vi "MQTT Subscriber.vi"() -> ()   [LabVIEW 2021]
uses:
  <vilib>/LabVIEW Open Source Project/MQTT Control Packets/Control Packets/CONNECT/ConnectFlags -- cluster.ctl
  <vilib>/LabVIEW Open Source Project/MQTT Client/Client class/Client.lvclass/Client.ctl
  <vilib>/LabVIEW Open Source Project/MQTT Client/Client class/Client.lvclass
  C:/Program Files (x86)/National Instruments/LabVIEW 2021/vi.lib/LabVIEW Open Source Project/MQTT Connection/MQTT_Base/Base Class/MQTT_Base.lvclass
  <vilib>/LabVIEW Open Source Project/Connection/Connection.TCP/Connection.TCP.lvclass
  C:/Program Files (x86)/National Instruments/LabVIEW 2021/vi.lib/LabVIEW Open Source Project/Connection/Connection/Connection.lvclass
  <vilib>/LabVIEW Open Source Project/MQTT Control Packets/Control Packets/PUBLISH/PUBLISH.lvclass
  <vilib>/LabVIEW Open Source Project/MQTT Connection/MQTT_Base/Base Class/MQTT_Base.lvclass
  <vilib>/LabVIEW Open Source Project/MQTT Control Packets/Control Packets/CONNECT/CONNECT.lvclass
panel:
  out "Connected?":bool
  out "Data Chart":dbl(graph)
  out "Data":dbl format="%#_4g"
  in  "Topic":string
  in  "remote port (1883)":u16=1883
  in  "address (localhost)":string="localhost"
  in  "STOP":bool
  # "MQTT Subscriber"
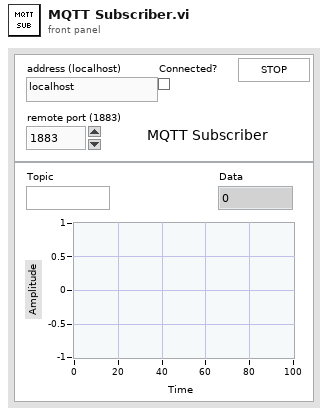
[diagram p1: front panel]
types:
  T1 = enum32{"Invalid", "Standard", "Closed", "Hidden", "Minimized", "Maximized"}
  T2 = enum32{"invalid app kind", "Development System", "Run Time System", "Student Edition", "Embedded LabVIEW", "Evaluation", "Custom"}
  T3 = cluster{"Will Topic":string, "Will Message":string, "Username":string, "Password":string}
  T4 = typedef "MQTT_Control_Packets.lvlib/CONNECT.lvclass/ConnectFlags -- cluster.ctl" = cluster{"Reserved":bool, "Clean Session":bool, "Will Flag":bool, "Will QoS 1":bool, "Will QoS 2":bool, "Will Retain":bool, "Password Flag":bool, "User Name Flag":bool}
  T5 = cluster{"Core":cluster{"Current VI Reference":refnum<vi>, "Close Panel on Exit?":bool}, "Connected?":bool}
  T6 = cluster{"Current VI Reference":refnum<vi>, "Close Panel on Exit?":bool}
  T7 = typedef "MQTT Client.lvlib/Client.lvclass/Public Events -- cluster.ctl" = cluster{"Connection Status":refnum<user-event>, "Connected":refnum<user-event>, "Application Message":refnum<user-event>}
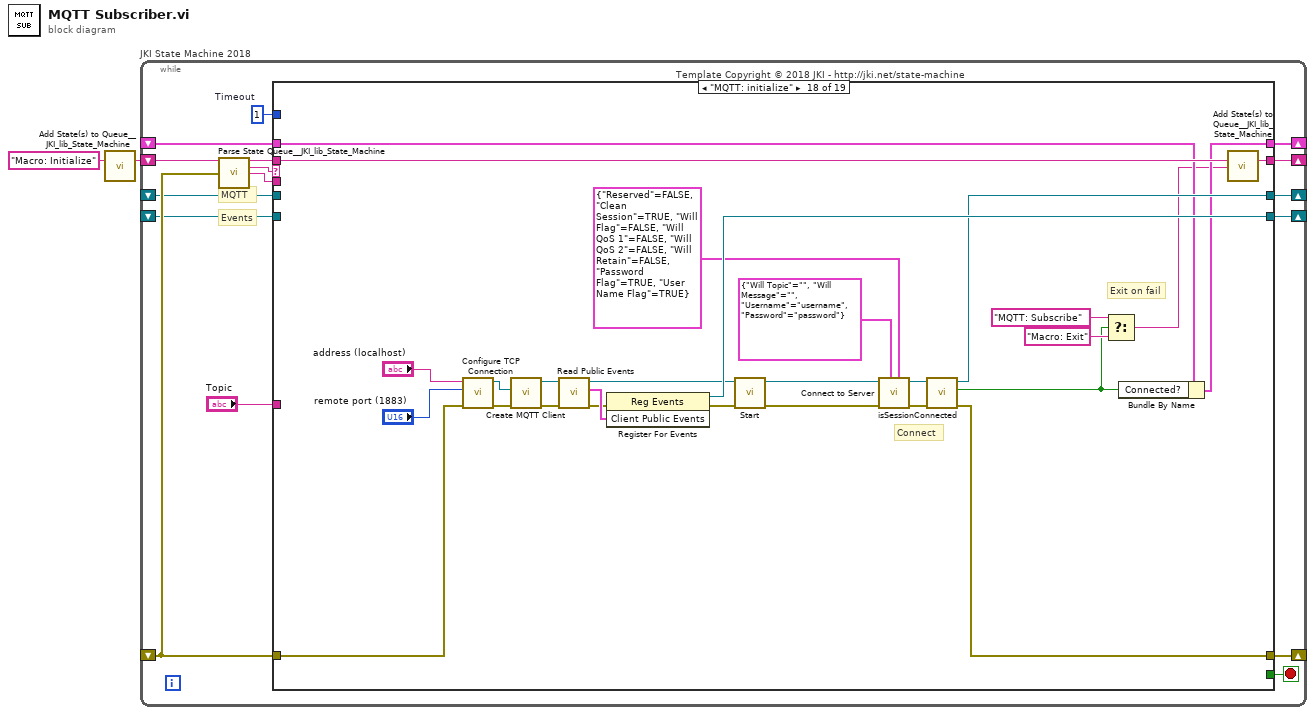
[diagram p0: block diagram]
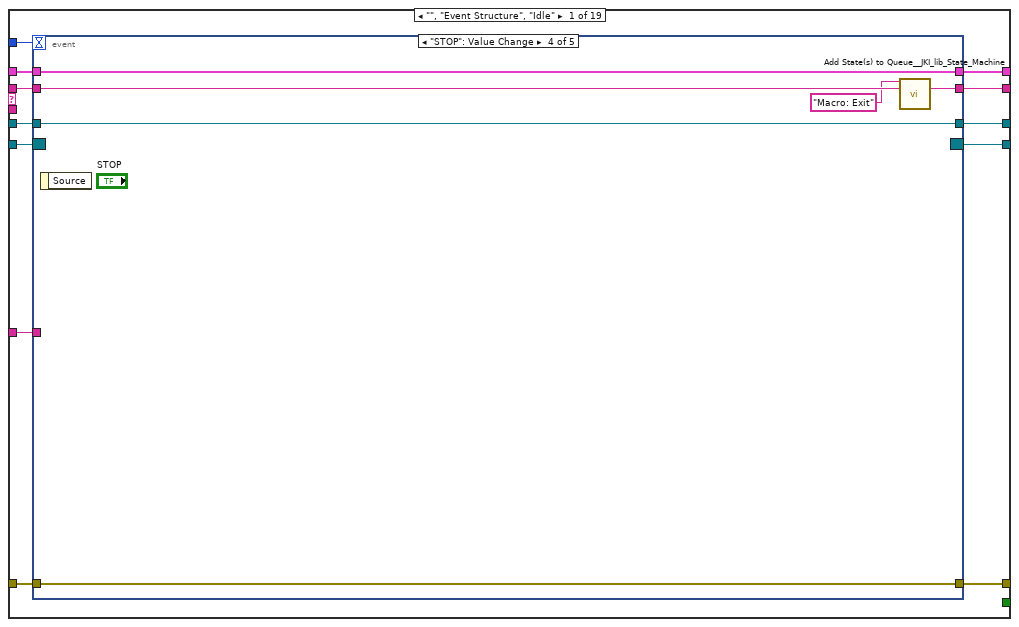
[diagram p2: hidden frame]
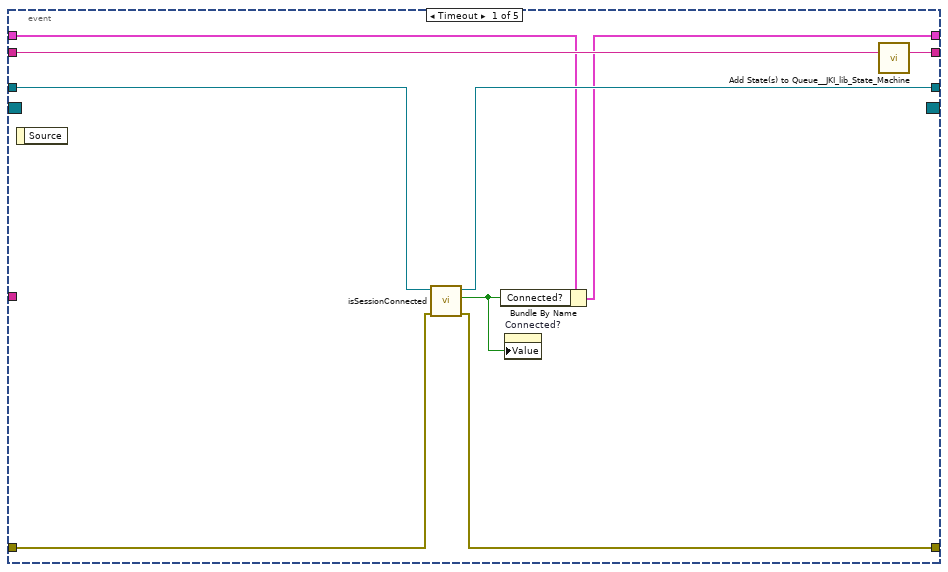
[diagram p3: hidden frame]
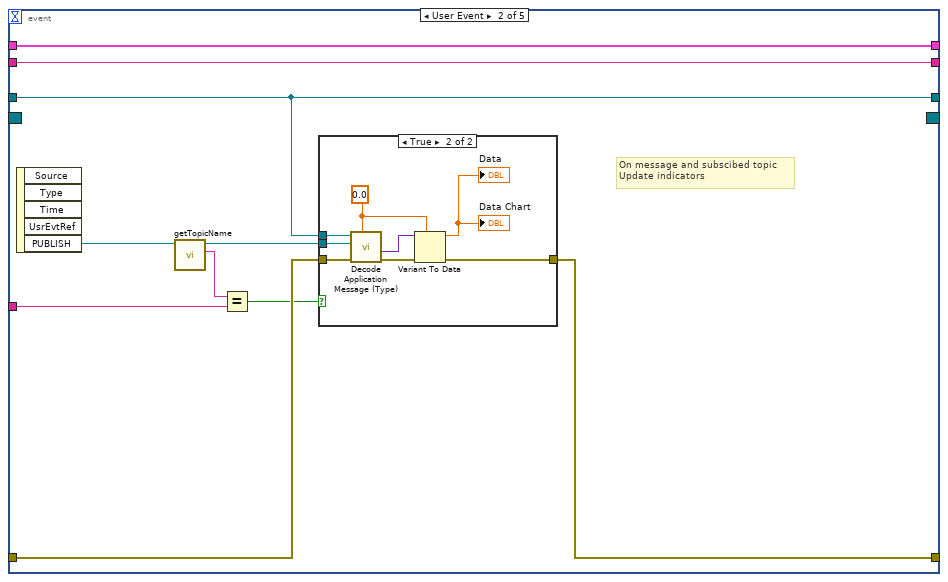
[diagram p4: hidden frame]
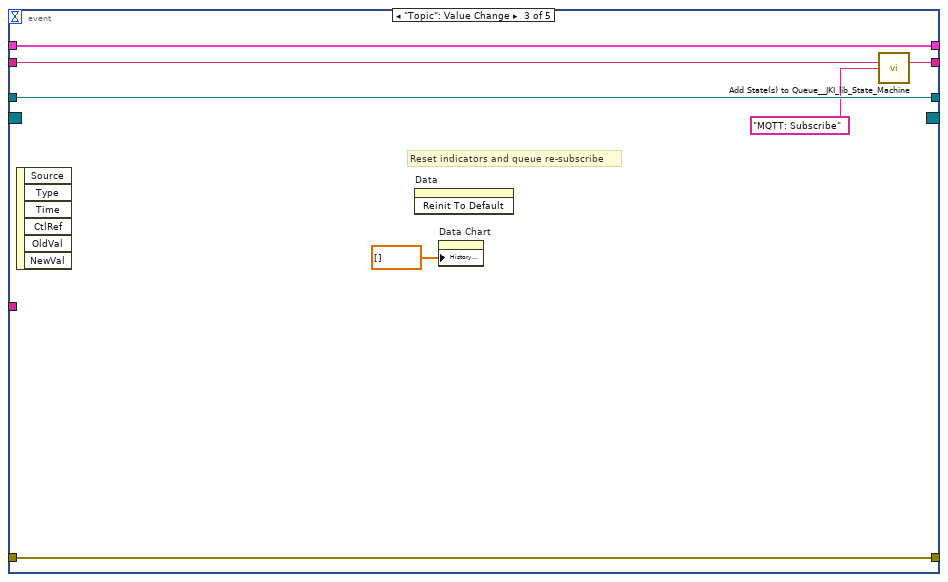
[diagram p6: hidden frame]
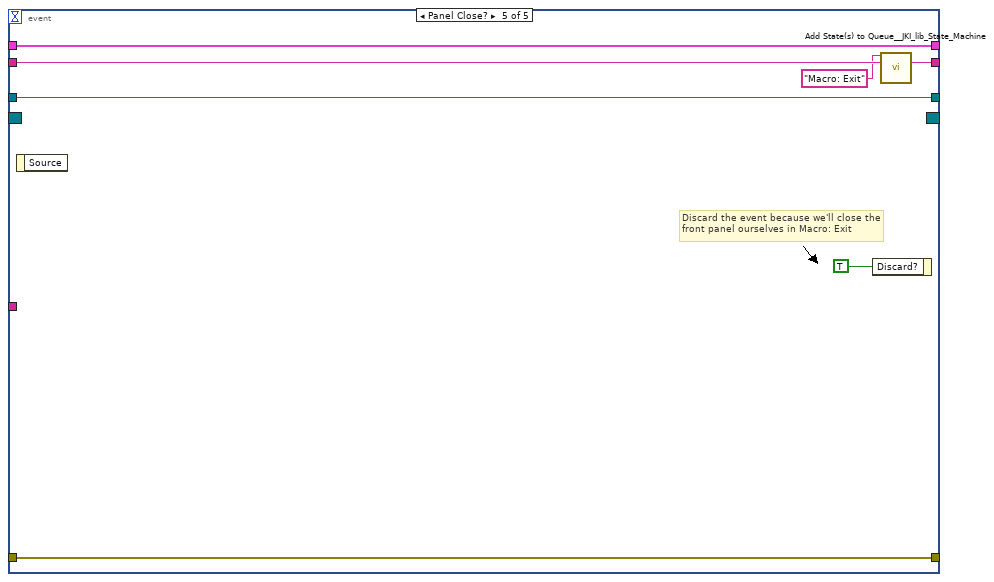
[diagram p7: hidden frame]
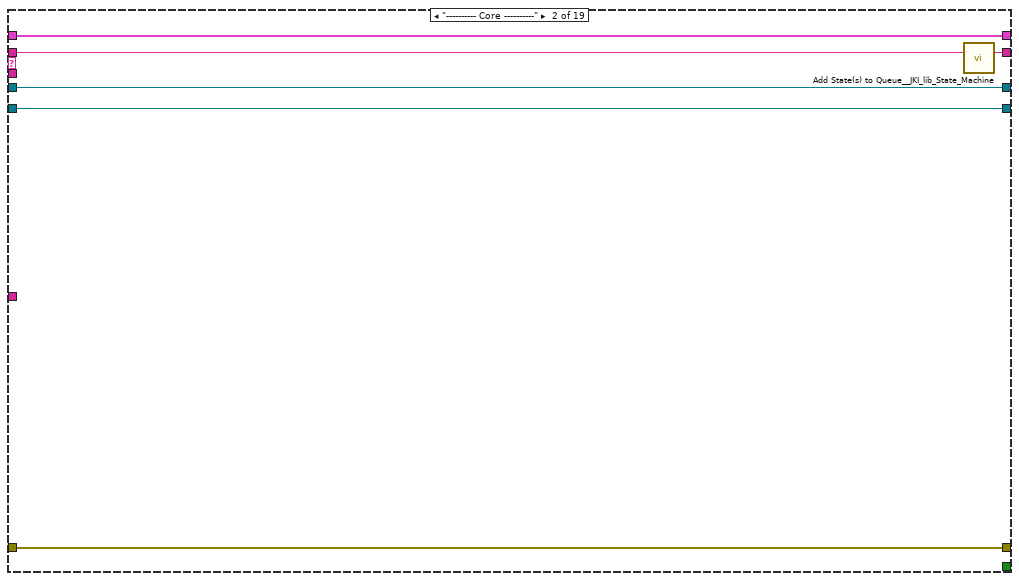
[diagram p8: hidden frame]
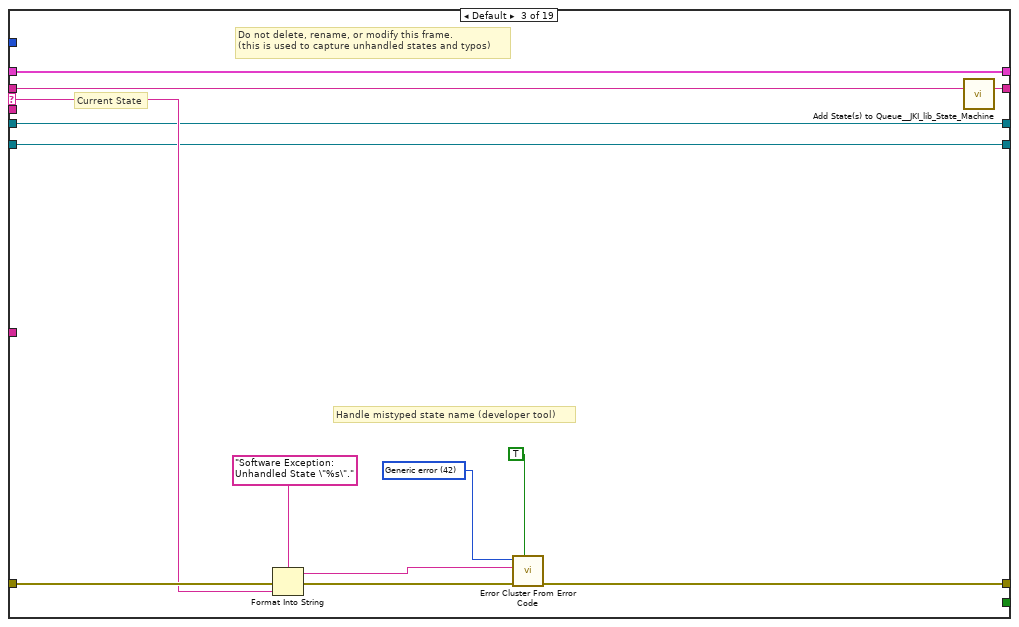
[diagram p9: hidden frame]
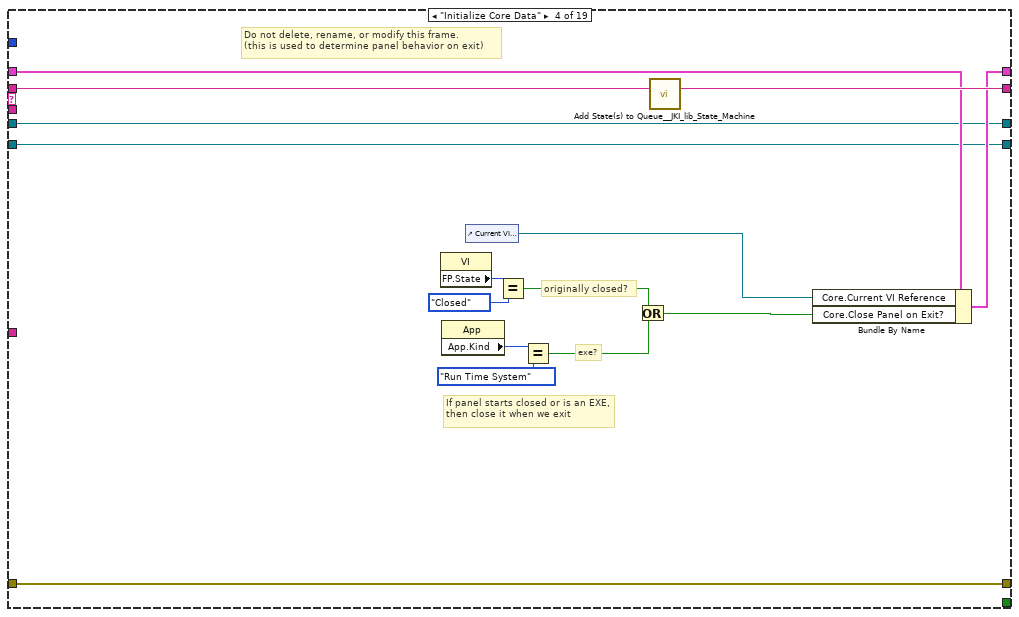
[diagram p10: hidden frame]
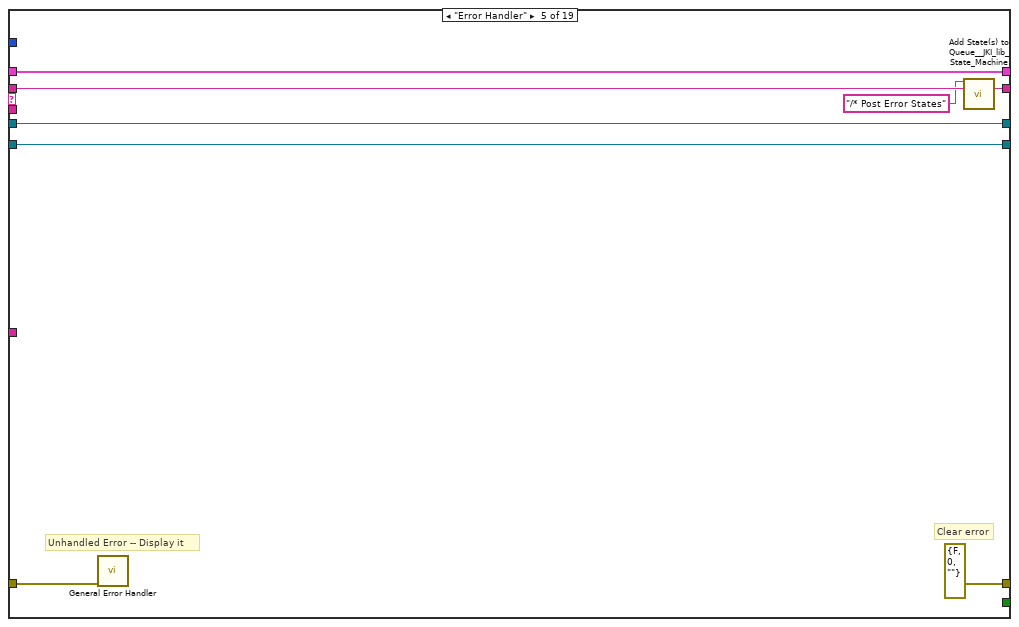
[diagram p11: hidden frame]
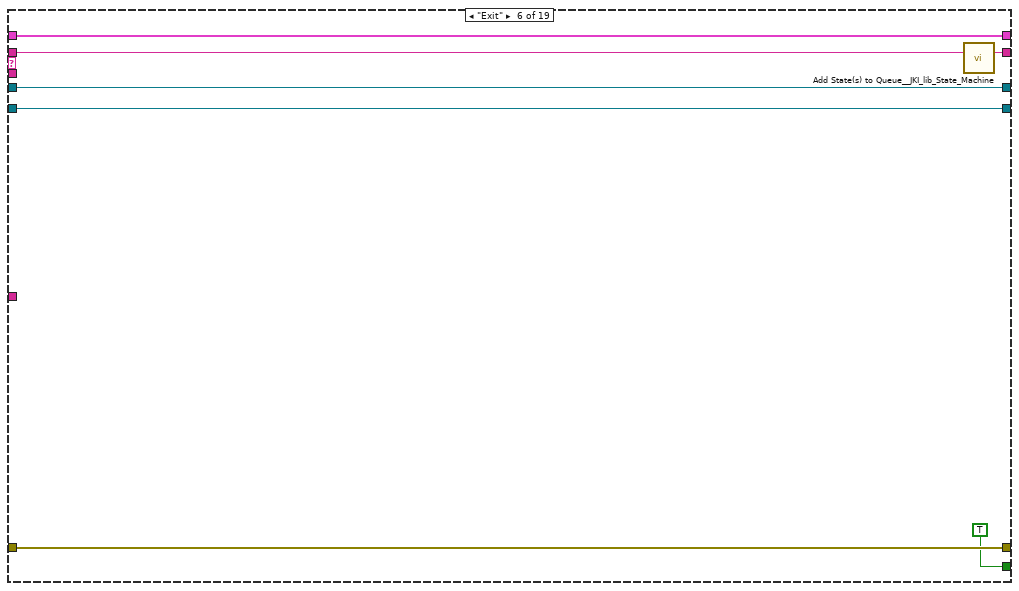
[diagram p12: hidden frame]
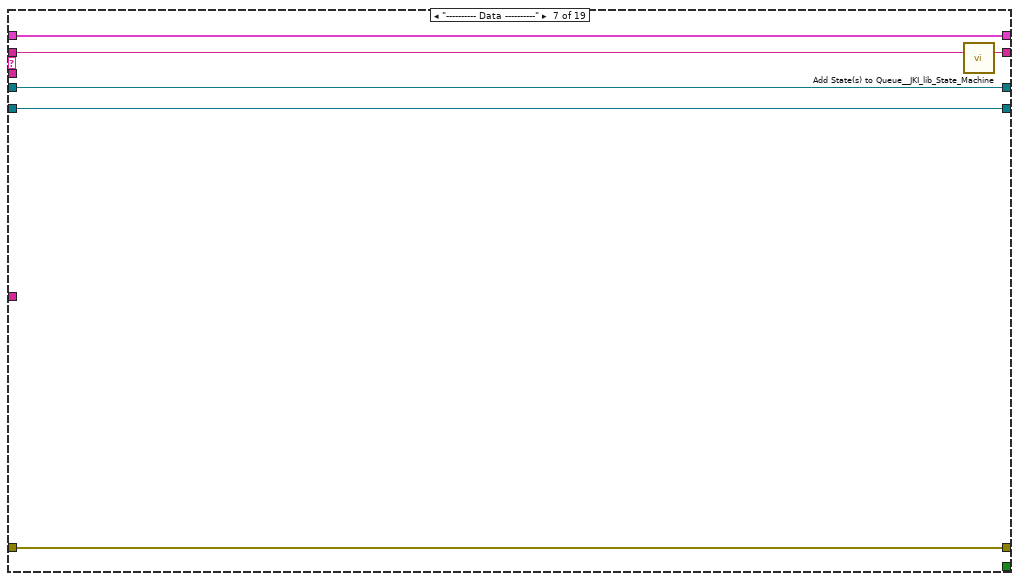
[diagram p13: hidden frame]
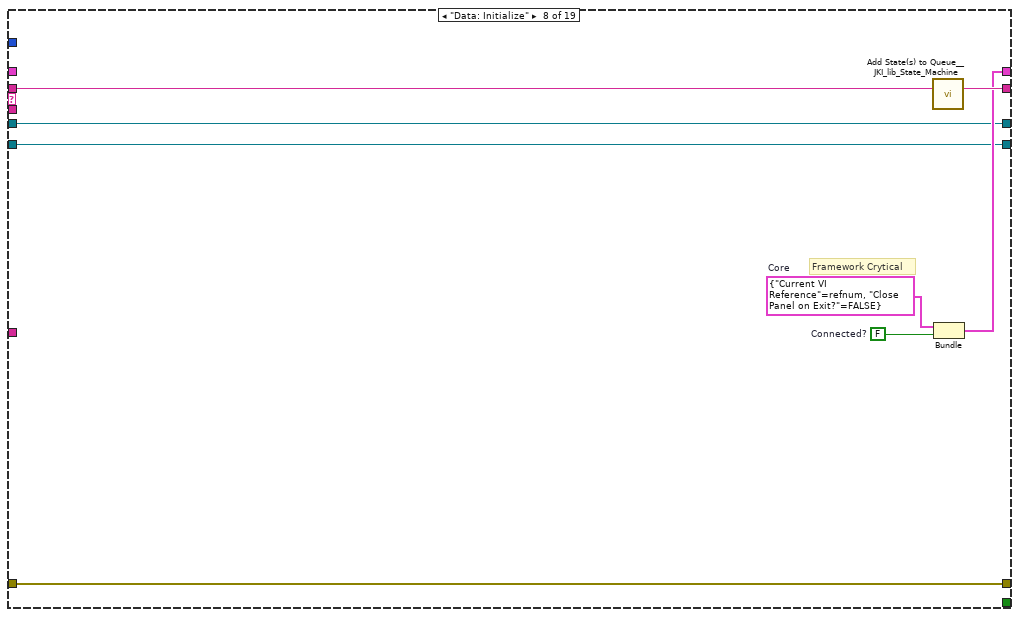
[diagram p14: hidden frame]
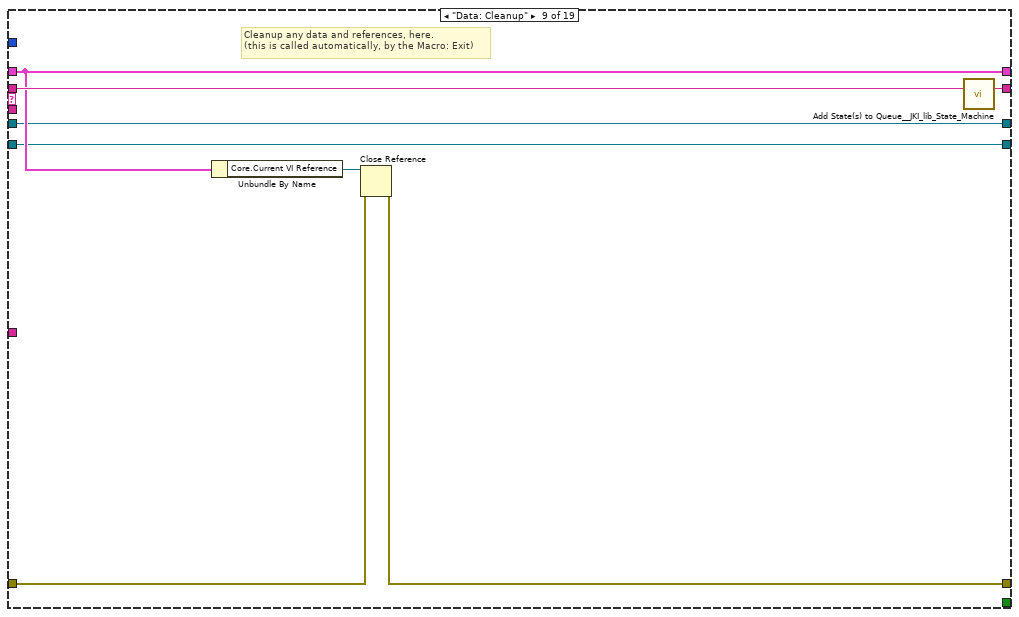
[diagram p15: hidden frame]
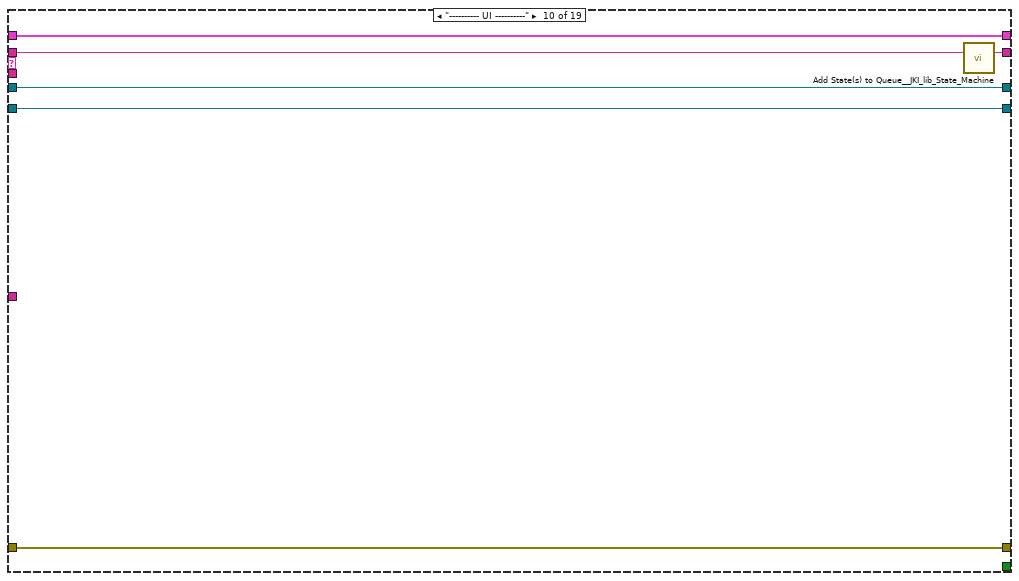
[diagram p16: hidden frame]
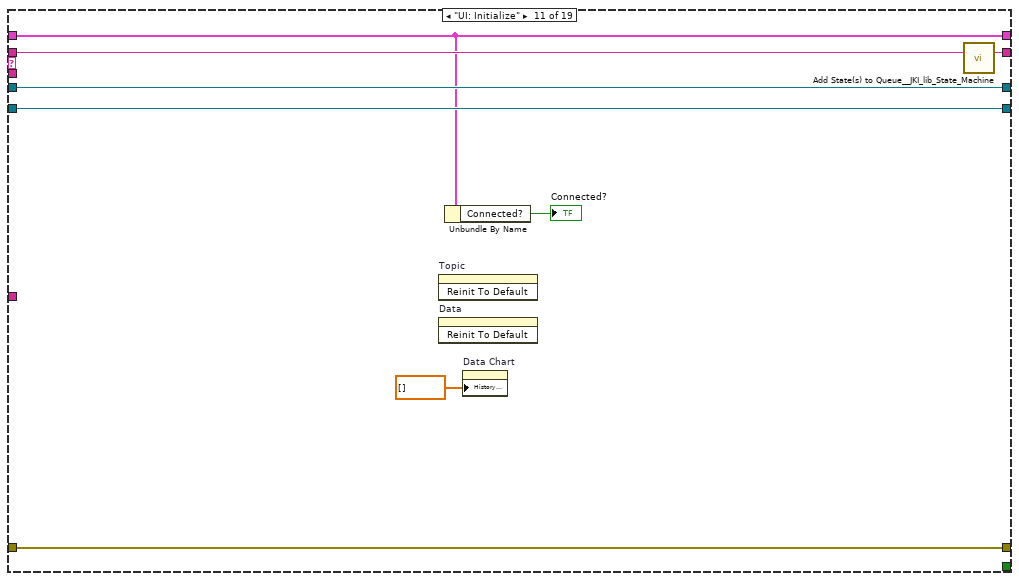
[diagram p17: hidden frame]
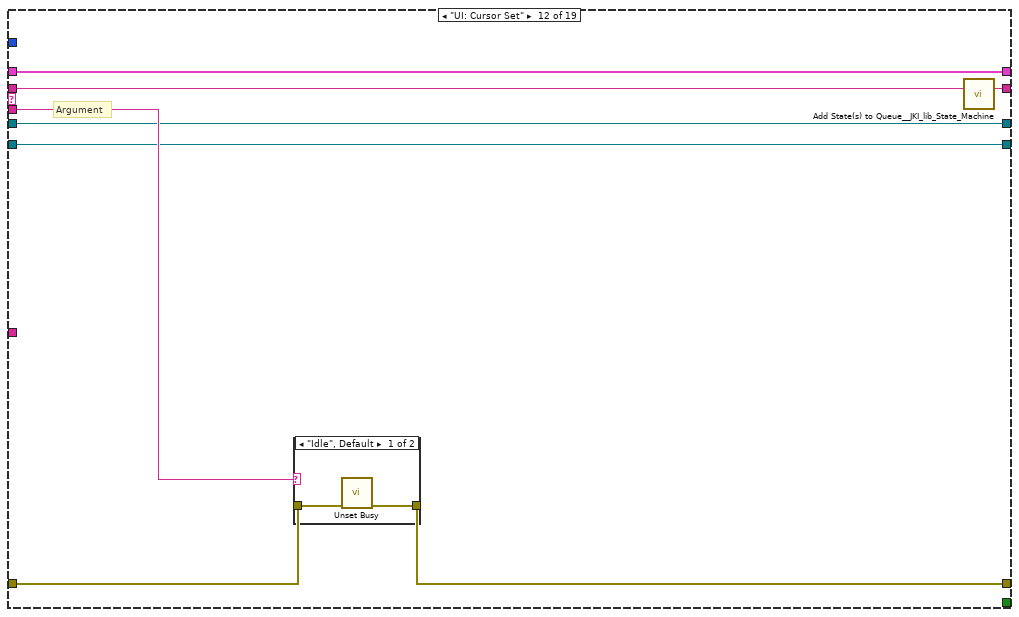
[diagram p18: hidden frame]
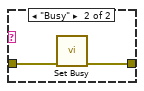
[diagram p19: hidden frame]
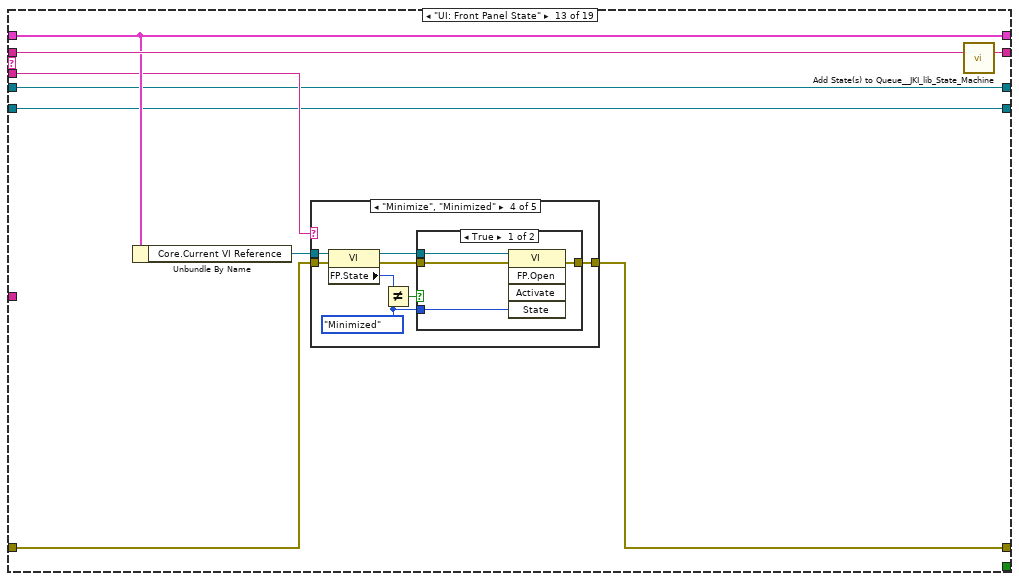
[diagram p20: hidden frame]
diagram:
  n1 = call <vilib>:"Add State(s) to Queue__JKI_lib_State_Machine.vi"("State(s) in (\"\")"="Macro: Initialize") -> ("States Out"=w2:string)  [unwired: 14 in]
  n2 = while "JKI State Machine 2018" {
    shift-right: [w11] -> _
    shift-left: _ -> [w10]
    shift-right: [w14] -> _
    shift-left: _ -> [w8]
    shift-right: [w13] -> _
    shift-left: w2 -> [w15]
    shift-right: [w7] -> _
    shift-left: _ -> [w6]
    shift-right: [w5] -> _
    shift-left: _ -> [w4]
    stop <- w12 stop-if-true
    w9 = 1  # Timeout
    # "Events"
    # "MQTT"
    # "Template Copyright © 2018 JKI - http://jki.net/state-machine"
    n3 = call <vilib>:"Parse State Queue__JKI_lib_State_Machine.vi"("State Queue"=w15, "Error In (no error)"=w8) -> ("Remaining States"=w17:string, "Current State"=w18:string, "Arguments"=w16:string)  [unwired: 11 in]
    n4 = case shown="\"MQTT: initialize\"" w18 {
      selector: w18 -> [_ _ w87 _ _ _ _ _ _ _ _ _ _ _ _ _ _ _ _]
      tunnel: w17 -> [w30 w84 w91 w112 w120 w127 w133 w141 w149 w155 w163 w171 w184 w255 w262 w274 w280 w308 w310]
      tunnel: w16 -> [_ _ _ _ _ _ _ _ _ _ _ w166 w178 _ _ _ _ _ _]
      tunnel: w10 -> [w28 w81 w89 w105 w117 w125 w130 _ w144 w152 w158 w169 w180 w252 w259 w271 w277 w288 w309]
      tunnel: [w27 w82 w93 w109 errorcluster {"status"=FALSE, "code"=0, "source"=""} ("error out") w124 w131 w138 w145 w153 w161 w167 w181 w253 w260 w272 w278 w290 w311] -> w14
      tunnel: w8 -> [w26 w82 w92 w109 w116 w124 w131 w138 w146 w153 w161 w168 w182 w253 w260 w272 w278 w306 w312]
      tunnel: [w29 w83 w90 w111 w119 w126 w132 w140 w148 w154 w162 w170 w183 w254 w261 w273 w279 w307 w310] -> w13
      tunnel: [_ _ _ _ _ TRUE _ _ _ _ _ _ _ _ _ _ _ _ _] -> w12
      tunnel: [w25 w81 w89 w110 w117 w125 w130 w139 w144 w152 w158 w169 w180 w252 w259 w271 w277 w287 w309] -> w11
      tunnel: w9 -> [w24 _ _ _ _ _ _ _ _ _ _ _ _ _ _ _ _ _ _]
      tunnel: [w20 w79 w85 w98 w113 w121 w128 w134 w142 w150 w159 w164 w176 w250 w256 w263 w275 w305 w319] -> w7
      tunnel: w6 -> [w21 w79 w85 w98 w113 w121 w128 w134 w142 w150 w159 w164 w176 w250 w256 w263 w275 _ w319]
      tunnel: [w22 w80 w86 w99 w114 w122 w129 w135 w143 w151 w160 w165 w177 w251 w257 w264 w276 w289 w313] -> w5
      tunnel: w4 -> [w23 w80 w86 w99 w114 w122 w129 w135 w143 w151 w160 w165 w177 w251 w257 w264 w276 _ w314]
      tunnel: "Topic" -> [w19 _ _ _ _ _ _ _ _ _ _ _ _ _ _ _ _ _ w315]
      frame "", "Event Structure", "Idle" {
        n5 = event shown="[3] \"STOP\": Value Change" {
          selector: w21 -> [_ _ _ _ _]
          dyn-events: [_ _ _ _ _] -> w20
          timeout: w24 -> [_ _ _ _ _]
          tunnel: w30 -> [w39 w49 w64 w71 w78]
          tunnel: [w38 w49 w63 w70 w77] -> w29
          tunnel: w28 -> [w33 w48 w65 w68 w75]
          tunnel: [w34 w42 w62 w69 w76] -> w27
          tunnel: w26 -> [w35 w43 w62 w69 w76]
          tunnel: [w32 w48 w65 w68 w75] -> w25
          tunnel: w23 -> [w37 w44 w61 w66 w72]
          tunnel: [w36 w44 w61 w66 w72] -> w22
          tunnel: w19 -> [_ w45 _ _ _]
          event Timeout {
            n6 = event-data() -> ()  [unwired: 1 in, 1 out]
            n7 = call <vilib>:"isSessionConnected.vi"("error in (no error)"=w35, "MQTT_Base in"=w37) -> ("error out"=w34:errorcluster, "Connected?"=w31:bool, "MQTT_Base out"=w36:refnum<class "Client.lvclass">)  [unwired: 7 in]
            n8 = Bundle By Name(cluster=w33, "Connected?"=w31) -> (w32:T5)
            n9 = property on="Connected?" class="Bool (strict)"("Value"=w31) -> ()  [unwired: 2 in, 2 out]
            n10 = call <vilib>:"Add State(s) to Queue__JKI_lib_State_Machine.vi"("State(s) in (\"\")"=w39) -> ("States Out"=w38:string)  [unwired: 14 in]
          }
          event User Event {
            # "On message and subscibed topic\nUpdate indicators"
            n11 = event-data() -> ("PUBLISH"=w47:refnum<class "PUBLISH.lvclass">)  [unwired: 1 in, 4 out]
            n12 = call <vilib>:"getTopicName.vi"("PUBLISH in"=w47) -> ("Topic"=w46:string, "PUBLISH out"=w40:refnum<class "PUBLISH.lvclass">)  [unwired: 8 in, 1 out]
            n13 = Equal?(x=w46, y=w45) -> (x = y?=w41:bool)
            n14 = case shown="True" w41 {
              tunnel: w44 -> [_ w58]
              tunnel: w43 -> [w50 w57]
              tunnel: [w50 w52] -> w42
              tunnel: w40 -> [_ w51]
              frame False {
              }
              frame True {
                w54 = 0.0
                n15 = call <vilib>:"Decode Application Message (Type).vi"("Type"=w54, "error in (no error)"=w57, "PUBLISH"=w51, "Client in"=w58) -> ("error out"=w55:errorcluster, "Payload"=w56:variant)  [unwired: 4 in, 2 out]
                n16 = Variant To Data(error in=w55, type=w54, Variant=w56) -> (data=→"Data" →"Data Chart":dbl, error out=w52:errorcluster)
              }
            }
          }
          event "Topic": Value Change {
            # "Reset indicators and queue re-subscribe"
            n17 = event-data() -> ()  [unwired: 1 in, 6 out]
            n18 = invoke on="Data" class="DigNum (strict)" method="Reinit To Default"() -> ()  [unwired: 3 in, 3 out]
            n19 = property on="Data Chart" class="WFChart (strict)"("History Data"=dbl[] []) -> ()  [unwired: 2 in, 2 out]
            n20 = call <vilib>:"Add State(s) to Queue__JKI_lib_State_Machine.vi"("State(s) in (\"\")"=w64, "State(s) at Back (\"\")"="MQTT: Subscribe" ("State(s) at Back (\"\")")) -> ("States Out"=w63:string)  [unwired: 13 in]
          }
          event "STOP": Value Change {
            n21 = event-data() -> ()  [unwired: 1 in, 1 out]
            n22 = call <vilib>:"Add State(s) to Queue__JKI_lib_State_Machine.vi"("State(s) in Front (\"\")"="Macro: Exit", "State(s) in (\"\")"=w71) -> ("States Out"=w70:string)  [unwired: 13 in]
          }
          event Panel Close? {
            # "Discard the event because we'll close the front panel ourselves in Macro: Exit"
            n23 = event-data() -> ()  [unwired: 1 in, 1 out]
            n24 = event-data("Discard?"=TRUE) -> ()  [unwired: 1 in, 1 out]
            n25 = call <vilib>:"Add State(s) to Queue__JKI_lib_State_Machine.vi"("State(s) in Front (\"\")"="Macro: Exit", "State(s) in (\"\")"=w78) -> ("States Out"=w77:string)  [unwired: 13 in]
          }
        }
      }
      frame "---------- Core ----------" {
        n26 = call <vilib>:"Add State(s) to Queue__JKI_lib_State_Machine.vi"("State(s) in (\"\")"=w84) -> ("States Out"=w83:string)  [unwired: 14 in]
      }
      frame Default {
        w96 = 42 items=["No error", "Argument error", "Memory is full", "Out of zone", "End of file", "File already open", "Generic file I/O error", "File not found", "File permission error", "Disk is full", "Duplicate path", "Too many files open", "System feature not enabled", "Resource file not found", "Cannot add resource", "Resource not found", "Image not found", "Image memory error", "Pen does not exist", "Config type invalid", "Config token not found", "Config parse error", "Config memory error", "Bad external code format", "Bad external code offset", "External code not present", "Null window", "Destroy window error", "Null menu", "Print aborted", "Bad print record", "Print driver error", "Windows error during printing", "Memory error during printing", "Print dialog error", "Generic print error", "Invalid device refnum", "Device not found", "Device parameter error", "Device unit error", "Cannot open device", "Device call aborted", "Generic error", "Cancelled by user", "Object ID too low", "Object ID too high", "Object not in heap", "Unknown heap", "Unknown object (invalid DefProc)", "Unknown object (DefProc not in table)", "Message out of range", "Invalid (null) method", "Unknown message", "Manager call not supported", "Bad address", "Network operation in progress", "Network operation timed out", "Connection is busy", "Network attribute not supported", "Network error", "Address in use", "System out of memory", "Connection aborted", "Connection refused", "Not connected", "Already connected", "Connection closed", "Initialization error (interapplication manager)", "Bad occurrence", "Wait on unbound occurrence handler", "Occurrence queue overflow", "Datalog type conflict", "Unused", "Unrecognized type (interapplication manager)", "Memory corrupt", "Failed to make temporary DLL", "Old CIN version", "Drag socket not found", "Failed to load drop-object", "Failed to register OLE object", "Failed to release OLE object", "Format specifier type mismatch", "Unknown format specifier", "Too few format specifiers", "Too many format specifiers", "Scan failed", "Newer CIN version", "Error converting to variant", "Runtime menu error", "Password tampered", "Variant attribute not found", "Incompatible variant data type", "Event data is not available", "Event Store is not present", "Occurrence is not found", "Event Queue is not created", "Event info is not available", "Refnum passed is NULL", "Error retrieving Class GUID", "Error retrieving CoClass GUID", "Error retrieving TypeLib GUID.", "Bad built application magic bytes.", "Specific driver is different from the specific driver associated with the Logical Name.", "There is no session opened to the class driver.", "Max Error", "MAX - Error with config objects", "MAX - Error loading configuration", "MAX - Group not supported"]
        # "Current State"
        # "Do not delete, rename, or modify this frame.\n(this is used to capture unhandled states and typos)"
        # "Handle mistyped state name (developer tool)"
        n27 = Format Into String(format string="Software Exception: Unhandled State \"%s\"." ("message"), error in=w92, w87) -> (resulting string=w95:string, error out=w94:errorcluster)  [unwired: 1 in]
        n28 = call <vilib>:"Error Cluster From Error Code.vi"("show call chain? (False)"=TRUE, "error in (no error)"=w94, "error message (\"\")"=w95, "error code (0)"=w96) -> ("error out"=w93:errorcluster)  [unwired: 5 in]
        n29 = call <vilib>:"Add State(s) to Queue__JKI_lib_State_Machine.vi"("State(s) in (\"\")"=w91) -> ("States Out"=w90:string)  [unwired: 14 in]
      }
      frame "Initialize Core Data" {
        # "Do not delete, rename, or modify this frame.\n(this is used to determine panel behavior on exit)"
        # "originally closed?"
        # "exe?"
        # "If panel starts closed or is an EXE, then close it when we exit"
        n30 = property class="VI"() -> ("FP.State"=w102:T1)  [unwired: 2 in, 2 out]
        n31 = property class="App"() -> ("App.Kind"=w108:T2)  [unwired: 2 in, 2 out]
        n32 = control-ref of="Current VI Reference"() -> (w103:refnum<vi>)
        n33 = Equal?(x=w102, y=T1."Closed" ("Front Panel Window:State")) -> (x = y?=w100:bool)
        n34 = Equal?(x=w108, y=T2."Run Time System" ("Application:Kind")) -> (x = y?=w106:bool)
        n35 = Or(x=w100, y=w106) -> (x .or. y?=w104:bool)
        n36 = call <vilib>:"Add State(s) to Queue__JKI_lib_State_Machine.vi"("State(s) in (\"\")"=w112) -> ("States Out"=w111:string)  [unwired: 14 in]
        n37 = Bundle By Name(cluster=w105, "Core.Current VI Reference"=w103, "Core.Close Panel on Exit?"=w104) -> (w110:T5)
      }
      frame "Error Handler" {
        # "Unhandled Error -- Display it"
        # "Clear error"
        n38 = call <vilib>:"General Error Handler.vi"("error in (no error)"=w116) -> ()  [unwired: 10 in, 5 out]
        n39 = call <vilib>:"Add State(s) to Queue__JKI_lib_State_Machine.vi"("State(s) in Front (\"\")"="/* Post Error States", "State(s) in (\"\")"=w120) -> ("States Out"=w119:string)  [unwired: 13 in]
      }
      frame "Exit" {
        n40 = call <vilib>:"Add State(s) to Queue__JKI_lib_State_Machine.vi"("State(s) in (\"\")"=w127) -> ("States Out"=w126:string)  [unwired: 14 in]
      }
      frame "---------- Data ----------" {
        n41 = call <vilib>:"Add State(s) to Queue__JKI_lib_State_Machine.vi"("State(s) in (\"\")"=w133) -> ("States Out"=w132:string)  [unwired: 14 in]
      }
      frame "Data: Initialize" {
        w136 = T6 {"Current VI Reference"=refnum, "Close Panel on Exit?"=FALSE}  # Core
        w137 = FALSE  # Connected?
        # "Framework Crytical"
        n42 = call <vilib>:"Add State(s) to Queue__JKI_lib_State_Machine.vi"("State(s) in (\"\")"=w141) -> ("States Out"=w140:string)  [unwired: 14 in]
        n43 = Bundle("Core"=w136, "Connected?"=w137) -> (w139:T5)  [unwired: 1 in]
      }
      frame "Data: Cleanup" {
        # "Cleanup any data and references, here.\n(this is called automatically, by the Macro: Exit)"
        n44 = Unbundle By Name(w144) -> ("Core.Current VI Reference"=w147:refnum<vi>)
        n45 = Close Reference(reference=w147, error in (no error)=w146) -> (error out=w145:errorcluster)
        n46 = call <vilib>:"Add State(s) to Queue__JKI_lib_State_Machine.vi"("State(s) in (\"\")"=w149) -> ("States Out"=w148:string)  [unwired: 14 in]
      }
      frame "---------- UI ----------" {
        n47 = call <vilib>:"Add State(s) to Queue__JKI_lib_State_Machine.vi"("State(s) in (\"\")"=w155) -> ("States Out"=w154:string)  [unwired: 14 in]
      }
      frame "UI: Initialize" {
        n48 = invoke on="Topic" class="Str" method="Reinit To Default"() -> ()  [unwired: 3 in, 3 out]
        n49 = invoke on="Data" class="DigNum (strict)" method="Reinit To Default"() -> ()  [unwired: 3 in, 3 out]
        n50 = Unbundle By Name(w158) -> ("Connected?"=→"Connected?":bool)
        n51 = property on="Data Chart" class="WFChart (strict)"("History Data"=dbl[] []) -> ()  [unwired: 2 in, 2 out]
        n52 = call <vilib>:"Add State(s) to Queue__JKI_lib_State_Machine.vi"("State(s) in (\"\")"=w163) -> ("States Out"=w162:string)  [unwired: 14 in]
      }
      frame "UI: Cursor Set" {
        # "Argument"
        n53 = case shown="\"Idle\", Default" w166 {
          tunnel: w168 -> [w173 w175]
          tunnel: [w172 w174] -> w167
          frame "Idle", Default {
            n54 = call <vilib>:"Unset Busy.vi"("error in (no error)"=w173) -> ("error out"=w172:errorcluster)  [unwired: 10 in]
          }
          frame "Busy" {
            n55 = call <vilib>:"Set Busy.vi"("error in (no error)"=w175) -> ("error out"=w174:errorcluster)  [unwired: 9 in, 1 out]
          }
        }
        n56 = call <vilib>:"Add State(s) to Queue__JKI_lib_State_Machine.vi"("State(s) in (\"\")"=w171) -> ("States Out"=w170:string)  [unwired: 14 in]
      }
      frame "UI: Front Panel State" {
        n57 = Unbundle By Name(w180) -> ("Core.Current VI Reference"=w179:refnum<vi>)
        n58 = case shown="\"Minimize\", \"Minimized\"" w178 {
          tunnel: w182 -> [w190 w205 w216 w229 w242]
          tunnel: [w192 w206 w218 w231 w244] -> w181
          tunnel: w179 -> [w191 w203 w217 w230 w243]
          frame "Open", "Standard", Default {
            w185 = T1."Standard" ("State")
            n59 = property class="VI"(reference=w191, error in=w190) -> (reference out=w188:refnum<vi>, error out=w189:errorcluster, "FP.State"=w187:T1)
            n60 = Not Equal?(x=w187, y=w185) -> (x != y?=w186:bool)
            n61 = case shown="True" w186 {
              tunnel: [w196 w198] -> w192
              tunnel: w189 -> [w195 w198]
              tunnel: w188 -> [w194 _]
              tunnel: w185 -> [w193 _]
              frame True {
                n62 = invoke class="VI" method="FP.Open"(reference=w194, error in=w195, "Activate"=TRUE, "State"=w193) -> (error out=w196:errorcluster)  [unwired: 1 in, 4 out]
              }
              frame False {
              }
            }
          }
          frame "Close", "Closed" {
            n63 = property class="VI"(reference=w203, error in=w205) -> (reference out=w202:refnum<vi>, error out=w204:errorcluster, "FP.State"=w200:T1)
            n64 = Not Equal?(x=w200, y=T1."Closed" ("Front Panel Window:State")) -> (x != y?=w199:bool)
            n65 = case shown="True" w199 {
              tunnel: [w207 w210] -> w206
              tunnel: w204 -> [w207 w209]
              tunnel: w202 -> [_ w208]
              frame False {
              }
              frame True {
                n66 = invoke class="VI" method="FP.Close"(reference=w208, error in=w209) -> (error out=w210:errorcluster)  [unwired: 1 in, 2 out]
              }
            }
          }
          frame "Hidden", "Hide" {
            w211 = T1."Hidden" ("State")
            n67 = property class="VI"(reference=w217, error in=w216) -> (reference out=w214:refnum<vi>, error out=w215:errorcluster, "FP.State"=w213:T1)
            n68 = Not Equal?(x=w213, y=w211) -> (x != y?=w212:bool)
            n69 = case shown="True" w212 {
              tunnel: [w222 w223] -> w218
              tunnel: w215 -> [w221 w223]
              tunnel: w214 -> [w220 _]
              tunnel: w211 -> [w219 _]
              frame True {
                n70 = invoke class="VI" method="FP.Open"(reference=w220, error in=w221, "State"=w219) -> (error out=w222:errorcluster)  [unwired: 2 in, 4 out]
              }
              frame False {
              }
            }
          }
          frame "Minimize", "Minimized" {
            w224 = T1."Minimized" ("State")
            n71 = property class="VI"(reference=w230, error in=w229) -> (reference out=w227:refnum<vi>, error out=w228:errorcluster, "FP.State"=w226:T1)
            n72 = Not Equal?(x=w226, y=w224) -> (x != y?=w225:bool)
            n73 = case shown="True" w225 {
              tunnel: [w235 w236] -> w231
              tunnel: w228 -> [w234 w236]
              tunnel: w227 -> [w233 _]
              tunnel: w224 -> [w232 _]
              frame True {
                n74 = invoke class="VI" method="FP.Open"(reference=w233, error in=w234, "State"=w232) -> (error out=w235:errorcluster)  [unwired: 2 in, 4 out]
              }
              frame False {
              }
            }
          }
          frame "Maximize", "Maximized" {
            w237 = T1."Maximized" ("State")
            n75 = property class="VI"(reference=w243, error in=w242) -> (reference out=w240:refnum<vi>, error out=w241:errorcluster, "FP.State"=w239:T1)
            n76 = Not Equal?(x=w239, y=w237) -> (x != y?=w238:bool)
            n77 = case shown="True" w238 {
              tunnel: [w248 w249] -> w244
              tunnel: w241 -> [w247 w249]
              tunnel: w240 -> [w246 _]
              tunnel: w237 -> [w245 _]
              frame True {
                n78 = invoke class="VI" method="FP.Open"(reference=w246, error in=w247, "State"=w245) -> (error out=w248:errorcluster)  [unwired: 2 in, 4 out]
              }
              frame False {
              }
            }
          }
        }
        n79 = call <vilib>:"Add State(s) to Queue__JKI_lib_State_Machine.vi"("State(s) in (\"\")"=w184) -> ("States Out"=w183:string)  [unwired: 14 in]
      }
      frame "---------- Macro ----------" {
        n80 = call <vilib>:"Add State(s) to Queue__JKI_lib_State_Machine.vi"("State(s) in (\"\")"=w255) -> ("States Out"=w254:string)  [unwired: 14 in]
      }
      frame "Macro: Initialize" {
        n81 = call <vilib>:"Add State(s) to Queue__JKI_lib_State_Machine.vi"("State(s) in Front (\"\")"="Data: Initialize\nInitialize Core Data\nMQTT: Initialize\nUI: Initialize\nUI: Front Panel State >> Open", "State(s) in (\"\")"=w262) -> ("States Out"=w261:string)  [unwired: 13 in]
      }
      frame "Macro: Exit" {
        n82 = Unbundle By Name(w271) -> ("Core.Close Panel on Exit?"=w270:bool)
        n83 = Select(t="UI: Front Panel State >> Close", s=w270, f="") -> (s? t:f=w267:string)
        n84 = call <vilib>:"Add State(s) to Queue__JKI_lib_State_Machine.vi"("State(s) in (\"\")"=w267, "State(s) at Back (\"\")"="Data: Cleanup\nExit") -> ("States Out"=w265:string)  [unwired: 13 in]
        n85 = call <vilib>:"Add State(s) to Queue__JKI_lib_State_Machine.vi"("State(s) in Front (\"\")"=w265, "State(s) in (\"\")"=w274) -> ("States Out"=w273:string)  [unwired: 13 in]
      }
      frame "---------- MQTT Broker ----------" {
        n86 = call <vilib>:"Add State(s) to Queue__JKI_lib_State_Machine.vi"("State(s) in (\"\")"=w280) -> ("States Out"=w279:string)  [unwired: 14 in]
      }
      frame "MQTT: initialize" {
        # "Exit on fail"
        # "Connect"
        n87 = call <vilib>:"Configure TCP Connection.vi"("error in (no error)"=w306, "remote port (80)"="remote port (1883)", "address (localhost)"="address (localhost)") -> ("error out"=w301:errorcluster, "Connection.TCP"=w300:refnum<class "Connection.TCP.lvclass">)  [unwired: 7 in]
        n88 = call <vilib>:"Create MQTT Client.vi"("error in (no error)"=w301, "Connection Configuration"=w300) -> ("error out"=w298:errorcluster, "Client out"=w299:refnum<class "Client.lvclass">)  [unwired: 8 in]
        n89 = call <vilib>:"Read Public Events.vi"("error in (no error)"=w298, "Client in"=w299) -> ("error out"=w296:errorcluster, "Client Public Events"=w297:T7, "Client out"=w295:refnum<class "Client.lvclass">)  [unwired: 7 in]
        n90 = register-events(error in=w296, w297) -> (reference out=w305:refnum<event-registration>, error out=w304:errorcluster)  [unwired: 1 in]
        n91 = call <vilib>:"Start.vi"("error in (no error)"=w304, "MQTT_Base in"=w295) -> ("error out"=w293:errorcluster, "MQTT_Base out"=w294:refnum<class "Client.lvclass">)  [unwired: 7 in, 1 out]
        n92 = call <vilib>:"Connect to Server.vi"("Connect Flags"=T4 {"Reserved"=FALSE, "Clean Session"=TRUE, "Will Flag"=FALSE, "Will QoS 1"=FALSE, "Will QoS 2"=FALSE, "Will Retain"=FALSE, "Password Flag"=TRUE, "User Name Flag"=TRUE}, "Payload"=T3 {"Will Topic"="", "Will Message"="", "Username"="username", "Password"="password"}, "error in (no error)"=w293, "Client in"=w294) -> ("error out"=w291:errorcluster, "Client out"=w292:refnum<class "Client.lvclass">)  [unwired: 4 in, 2 out]
        n93 = call <vilib>:"isSessionConnected.vi"("error in (no error)"=w291, "MQTT_Base in"=w292) -> ("error out"=w290:errorcluster, "Connected?"=w284:bool, "MQTT_Base out"=w289:refnum<class "Client.lvclass">)  [unwired: 7 in]
        n94 = Select(t="MQTT: Subscribe", s=w284, f="Macro: Exit" ("State(s) at Back (\"\")")) -> (s? t:f=w283:string)
        n95 = Bundle By Name(cluster=w288, "Connected?"=w284) -> (w287:T5)
        n96 = call <vilib>:"Add State(s) to Queue__JKI_lib_State_Machine.vi"("State(s) in (\"\")"=w308, "State(s) at Back (\"\")"=w283) -> ("States Out"=w307:string)  [unwired: 13 in]
      }
      frame "MQTT: Subscribe" {
        n97 = call <vilib>:"isSessionConnected.vi"("error in (no error)"=w312, "MQTT_Base in"=w314) -> ("error out"=w317:errorcluster, "Connected?"=w316:bool, "MQTT_Base out"=w318:refnum<class "Client.lvclass">)  [unwired: 7 in]
        n98 = case shown="True" w316 {
          tunnel: w318 -> [w321 w326]
          tunnel: w317 -> [w320 w325]
          tunnel: [w320 w324] -> w311
          tunnel: [w321 w323] -> w313
          tunnel: w315 -> [_ w322]
          frame False {
          }
          frame True {
            n99 = call <vilib>:"Subscribe (Scalar).vi"("error in (no error)"=w325, "Topic Filter"=w322, "Client in"=w326) -> ("error out"=w324:errorcluster, "Client out"=w323:refnum<class "Client.lvclass">)  [unwired: 6 in, 1 out]
          }
        }
        n100 = property on="Connected?" class="Bool (strict)"("Value"=w316) -> ()  [unwired: 2 in, 2 out]
      }
    }
  }
